vi "Double FFT Mesurament RT.vi"() -> ()   [LabVIEW 2014]
uses:
  <vilib>/Platform/TimedLoop/XDataNode/timing_clust.ctl
  <vilib>/Platform/TimedLoop/XDataNode/nitl_modes.ctl
  <vilib>/Platform/TimedLoop/XDataNode/wakeup.ctl
  <vilib>/FPGAPlugInAG/sbRIO-9636/niLvFpga_Open_sbRIO-9636.vi
  <vilib>/rvi/interface/common/dynamic/niFpgaDynamicAddResources.vi
  <vilib>/Utility/error.llb/Error Cluster From Error Code.vi
  <vilib>/rvi/errors/niLvFpgaAdjustHostInterfaceError.vi
  <vilib>/rvi/interface/common/niFpgaWaitOnOcc.vi
  <vilib>/FPGAPlugInAG/Dynamic/niLvFpga_Run_Dynamic.vi
  <vilib>/FPGAPlugInAG/Dynamic/niLvFpga_Abort_Dynamic.vi
  <vilib>/FPGAPlugInAG/Dynamic/niLvFpga_Reset_Dynamic.vi
  <vilib>/FPGAPlugInAG/Dynamic/niLvFpga_Close_Dynamic.vi
  <vilib>/rvi/interface/nirviOpenFPGA/nirviOpenFPGA.xnode
  FPGA Bitfiles/LaserDistanceSen_FPGATarget_DoubleFFTMesuram_r82pz3ZO4sk.lvbitx
  FPGA Target/Test VIs/Double FFT Mesurament Test.vi
  FPGA Bitfiles/LaserDistanceSen_FPGATarget_DoubleFFTMesuram_atjrRfXVdPQ.lvbitx
  FPGA Target/Test VIs/Double FFT Mesurament Test SLOW.vi
  <vilib>/rvi/interface/nirviReadWriteControl/nirviReadWriteControl.xnode
  <vilib>/rvi/interface/nirviMethod/nirviMethod.xnode
  <vilib>/Platform/TimedLoop/XDataNode/XDataNode.xnode
  <vilib>/rvi/interface/nirviCloseFPGA/nirviCloseFPGA.xnode
  <vilib>/FPGAPlugInAG/Dynamic/niLvFpga_ConfigureFifo_Dynamic.vi
  <vilib>/rvi/errors/niLvFpgaMergeErrorWithErrorCode.vi
  <vilib>/FPGAPlugInAG/Dynamic/niLvFpga_StartFifo_Dynamic.vi
  <vilib>/rvi/interface/Simulation/niFpgaSimulationCallBeginRW.vi
  <vilib>/FPGAPlugInAG/Dynamic/niLvFpga_ReadFifo_Dynamic.vi
  <vilib>/Platform/TimedLoop/XDataNode/XDNodeRunTimeDep.lvlib
  NiFpgaLv.dll
panel:
  in  "Sample /Modulation Frequency":enum32{"40MHz/32KHz", "30MHz/24Khz"}(radio)
  out "Det Freq 1 (3-point) 2":dbl(graph)
  out "Det Freq 1":dbl(graph)
  out "Det Freq 2":T1(graph)
  out "Det Freq 2 (3-point)":dbl(graph)
  out "Detected Frequency (Hz) 1 (3-point)":dbl
  out "Detected Frequency (Hz) 2 (3-point)":dbl
  in  "Scale factor":dbl=1.0 format="%#_13g"
  out "Mean Noise 2":dbl
  out "Mean Noise 1":dbl
  in  "tieni premuto per":i32=1
  out "Mean Frequency":dbl
  out "Velocity (m/s)":dbl
  out "Distance (m)":dbl
  in  "Triangolo dritto?":bool
  out "Detected Frequency (Hz) 2":dbl
  out "Detected Frequency (Hz) 1":dbl
  out "Interpolate Bin 2":dbl
  out "Interpolate Bin 1":dbl
  out "Check Delta Amp Ok? 2":bool
  out "Check Delta Amp Ok? 1":bool
  out "Delta difference % 2":dbl
  out "Delta difference % 1":dbl
  in  "Max Delta Difference bin % 2":dbl=10.0
  in  "Max Delta Difference bin % 1":dbl=10.0
  out "Check Amp 2 Ok?":bool
  out "Check Amp Ok?":bool
  in  "Threshold Amp 2":dbl=5500.0
  in  "Threshold Amp 1":dbl=5500.0
  out "Prev Max Bin 2":i32
  out "Max Bin 2":i32
  out "Succ Max Bin 2":i32
  out "Prev Max Amp 2":dbl
  out "Max Amp 2":dbl
  out "Succ Max Amp 2":dbl
  out "Succ Max Amp":dbl
  out "Max Amp":dbl
  out "Prev Max Amp":dbl
  out "Succ Max Bin":i32
  out "Max Bin":i32
  out "Prev Max Bin":i32
  in  "stop":bool
  in  "Initial Latency points":u32(slide) scale=0.0..1249.0
  out "Second FFT (bin)":dbl[](graph)
  out "Second Signal (points) - Rising Triangular":dbl[](graph)
  out "Elements Remaining FFT":u32
  out "Elements Remaining Signal":u32
  out "First FFT (bin)":dbl[](graph)
  out "First Signal (points) - Falling Triangular":dbl[](graph)
  in  "Snapshot":bool
  in  "Windowing":T2(ring)
  in  "first bin":i32=5
  in  "last bin":i32=255
  in  "lower limit 2":u32(slide)=738 scale=625.0..738.0
  in  "lower limit 1":u32(slide)=113 scale=0.0..113.0
  # "OFFLINE parameters"
  # "WARNING:\nOnce pressed wait untill the end of operation"
  # "Max Detection FFT bin range"
  # "Bin \nDetection"
  # "(2*Max_rumore=2*2700)"
  # "Bin Amplitude\n      CHECK"
  # "(2*Max_rumore=2*2700)"
  # "Bin difference\n     CHECK"
  # "Bin interpolation"
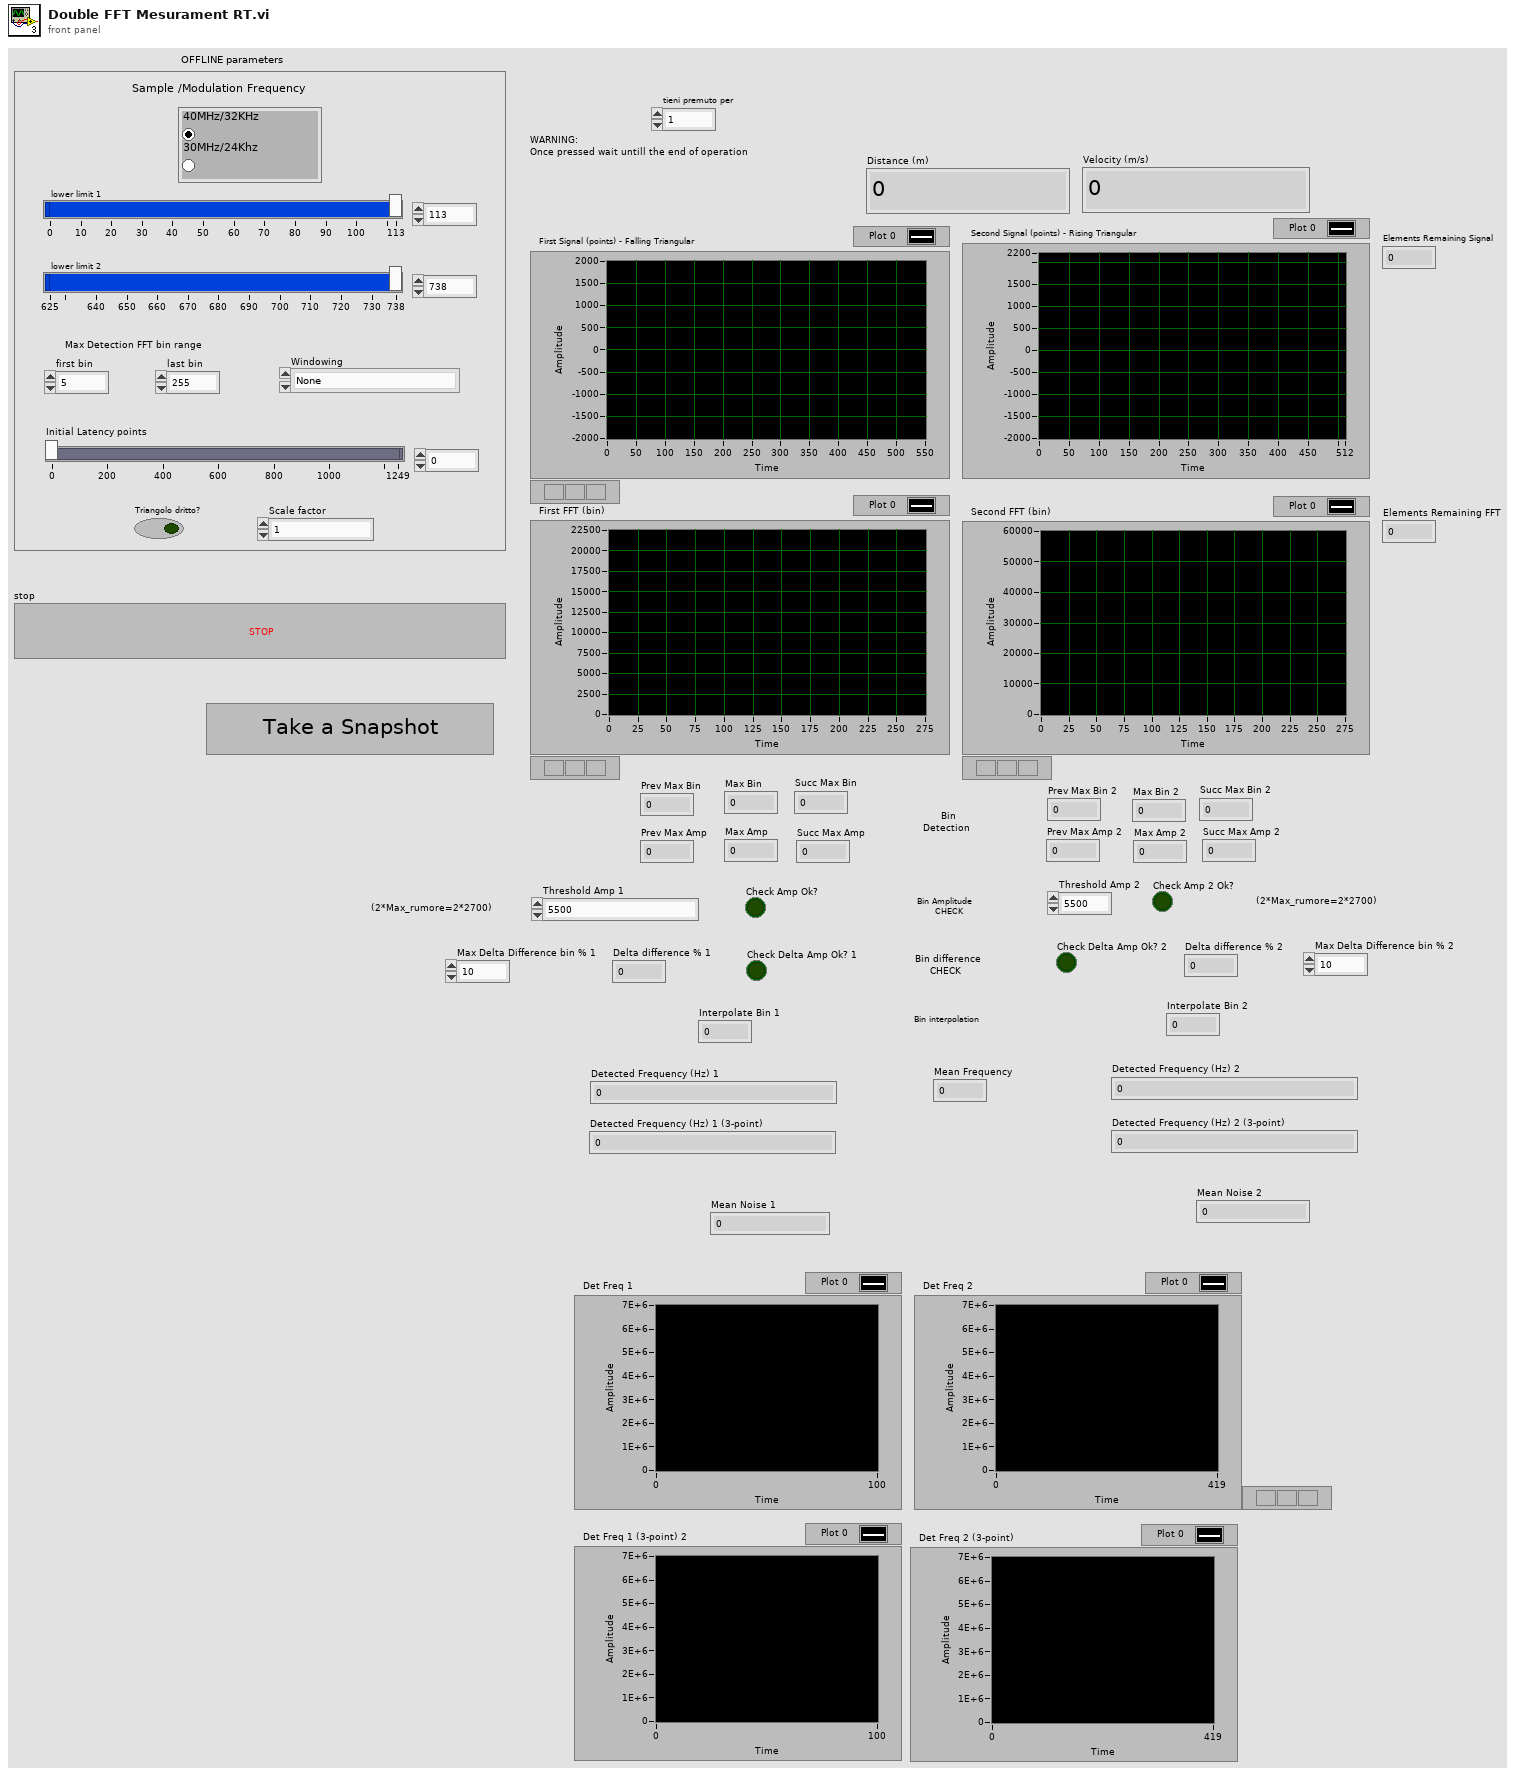
[diagram p1: front panel]
types:
  T1 = cluster{"Delta difference %":dbl, "Detected Frequency (Hz)":dbl}
  T2 = enum16{"None", "Hanning", "Hamming", "Blackman", "Blackman-Harris"}
  T3 = typedef "XDNodeRunTimeDep.lvlib/timing_clust.ctl" = cluster{"Expected End [f-1]":u64, "Actual End [f-1]":u64, "Finished Late? [f-1]":bool, "Expected End [i-1]":u64, "Actual End [i-1]":u64, "Finished Late? [i-1]":bool, "Expected Start [i]":u64, "Actual Start [i]":u64, "Expected Start [f]":u64, "Actual Start [f]":u64, "Source Name":string, "Structure Name":string, "Period":i64, "Deadline":i64, "Offset":i64, "Start":i64, "Priority":i32, "Timeout":i32, "Mode":T4, "Wakeup Reason":T5, "Error":errorcluster, "Source Type":string, "Secondary Source Type":string, "Global End Time":u64, "Global Start Time":u64, "Frame Duration":u64, "Iteration Duration":u64, "Assigned CPU":i32, "I/O Scan Engine Mode":u32}
  T4 = typedef "XDNodeRunTimeDep.lvlib/nitl_modes.ctl" = enum32{"No Change", "Process missed periods, maintain original phase", "Discard missed periods, maintain original phase", "Process missed periods, ignore original phase", "Discard missed periods, ignore original phase"}
  T5 = typedef "XDNodeRunTimeDep.lvlib/wakeup.ctl" = enum32{"Normal", "Aborted", "Asynchronous wakeup", "Timing source error", "Timed loop error", "Timeout"}
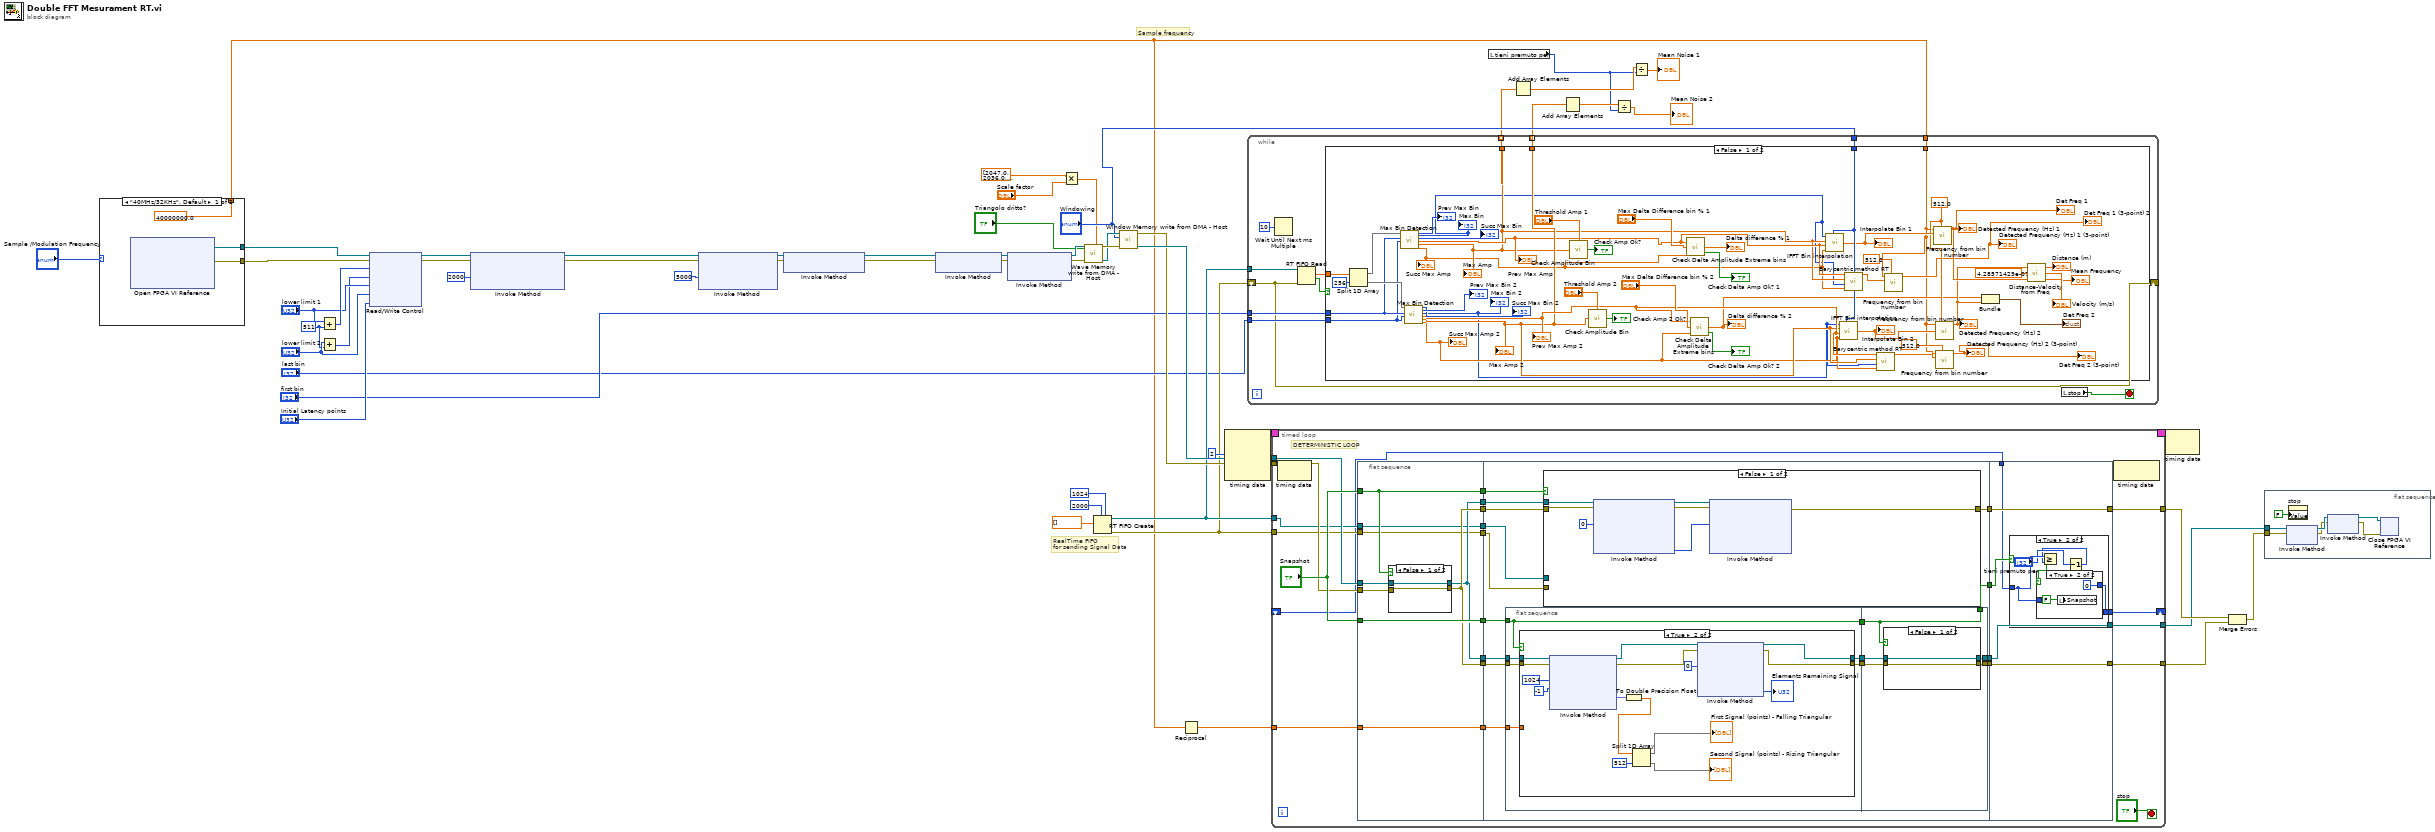
[diagram p0: block diagram]
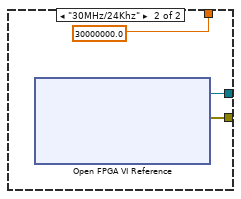
[diagram p2: hidden frame]
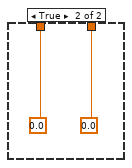
[diagram p3: hidden frame]
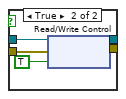
[diagram p4: hidden frame]
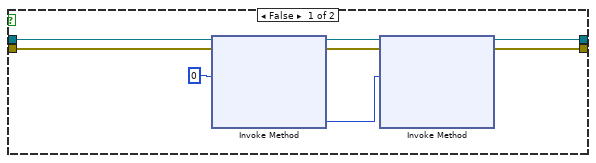
[diagram p5: hidden frame]
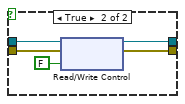
[diagram p6: hidden frame]
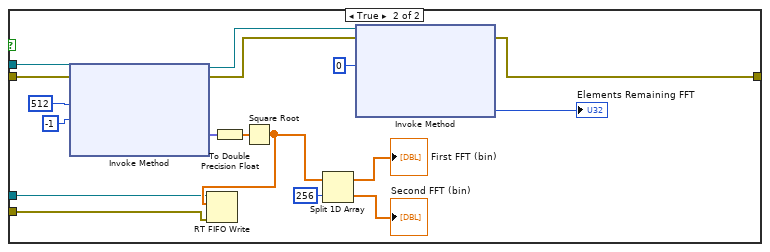
[diagram p7: hidden frame]
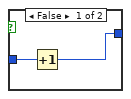
[diagram p9: hidden frame]
diagram:
  w51 = u32 511 ("y")
  # "Sample frequency"
  # "RealTime FIFO \nfor sending Signal Data"
  n1 = case shown="\"40MHz/32KHz\", Default" "Sample /Modulation Frequency" {
    tunnel: [w58 w61] -> w50
    tunnel: [w57 w60] -> w49
    tunnel: [40000000.0 30000000.0] -> w1
    frame "40MHz/32KHz", Default {
      n2 = xnode "Open FPGA VI Reference"() -> ("FPGA VI Reference Out"=w58:refnum<k20>, "error out"=w57:errorcluster)  [unwired: 2 in]
    }
    frame "30MHz/24Khz" {
      n3 = xnode "Open FPGA VI Reference"() -> ("FPGA VI Reference Out"=w61:refnum<k20>, "error out"=w60:errorcluster)  [unwired: 2 in]
    }
  }
  n4 = Add(x="lower limit 1", y=w51) -> (x+y=w55:u32)
  n5 = Add(x="lower limit 2", y=w51) -> (x+y=w53:u32)
  n6 = xnode "Read/Write Control"("FPGA VI Reference In"=w50, "error in"=w49, "upper limit 1"=w55, "upper limit 2"=w53, "lower limit 1"="lower limit 1", "lower limit 2"="lower limit 2", "Latency points"="Initial Latency points") -> ("FPGA VI Reference Out"=w46:refnum<k20>, "error out"=w45:errorcluster)
  n7 = xnode "Invoke Method"("FPGA VI Reference In"=w46, "error in"=w45, "Requested Depth"=u32 2000) -> ("FPGA VI Reference Out"=w24:refnum<k20>, "error out"=w25:errorcluster)  [unwired: 1 out]
  n8 = xnode "Invoke Method"("FPGA VI Reference In"=w24, "error in"=w25, "Requested Depth"=u32 5000) -> ("FPGA VI Reference Out"=w36:refnum<k20>, "error out"=w37:errorcluster)  [unwired: 1 out]
  n9 = xnode "Invoke Method"("FPGA VI Reference In"=w36, "error in"=w37) -> ("FPGA VI Reference Out"=w22:refnum<k20>, "error out"=w23:errorcluster)
  n10 = xnode "Invoke Method"("FPGA VI Reference In"=w22, "error in"=w23) -> ("FPGA VI Reference Out"=w34:refnum<k20>, "error out"=w35:errorcluster)
  n11 = xnode "Invoke Method"("FPGA VI Reference In"=w34, "error in"=w35) -> ("FPGA VI Reference Out"=w40:refnum<k20>, "error out"=w39:errorcluster)  [unwired: 1 in]
  n12 = Multiply(x=dbl[] [2047.0, 2036.0, 2024.0, 2013.0, 2002.0, 1990.0, 1979.0, 1968.0, 1956.0, 1945.0, 1934.0, 1923.0, 1912.0, 1900.0, 1889.0, 1878.0, 1867.0, 1856.0, 1845.0, 1833.0, 1822.0, 1811.0, 1800.0, 1789.0, 1778.0, 1767.0, 1756.0, 1745.0, 1734.0, 1723.0, 1712.0, 1702.0, 1691.0, 1680.0, 1669.0, 1658.0, 1647.0, 1636.0, 1626.0, 1615.0, 1604.0, 1593.0, 1583.0, 1572.0, 1561.0, 1550.0, 1540.0, 1529.0, 1518.0, 1508.0, 1497.0, 1487.0, 1476.0, 1465.0, 1455.0, 1444.0, 1434.0, 1423.0, 1413.0, 1402.0, 1392.0, 1381.0, 1371.0, 1360.0, 1350.0, 1340.0, 1329.0, 1319.0, 1309.0, 1298.0, 1288.0, 1278.0, 1267.0, 1257.0, 1247.0, 1237.0, 1226.0, 1216.0, 1206.0, 1196.0, 1186.0, 1176.0, 1165.0, 1155.0, 1145.0, 1135.0, 1125.0, 1115.0, 1105.0, 1095.0, 1085.0, 1075.0, 1065.0, 1055.0, 1045.0, 1035.0, 1025.0, 1015.0, 1006.0, 996.0, 986.0, 976.0, 966.0, 956.0, 947.0, 937.0, 927.0, 917.0, 908.0, 898.0, 888.0, 879.0, 869.0, 859.0, 850.0, 837.0, 826.0, 816.0, 804.0, 796.0, 788.0, 778.0, 769.0, 758.0, 750.0, 743.0, 733.0, 724.0, 717.0, 709.0, 701.0, 693.0, 686.0, 677.0, 669.0, 661.0, 653.0, 645.0, 638.0, 630.0, 622.0, 615.0, 607.0, 599.0, 592.0, 583.0, 576.0, 569.0, 561.0, 554.0, 547.0, 539.0, 532.0, 525.0, 518.0, 509.0, 501.0, 492.0, 486.0, 478.0, 471.0, 463.0, 456.0, 450.0, 442.0, 435.0, 429.0, 421.0, 415.0, 408.0, 401.0, 394.0, 388.0, 381.0, 375.0, 368.0, 361.0, 355.0, 349.0, 342.0, 336.0, 330.0, 323.0, 317.0, 311.0, 304.0, 298.0, 292.0, 286.0, 279.0, 273.0, 267.0, 261.0, 255.0, 249.0, 242.0, 236.0, 230.0, 224.0, 218.0, 212.0, 206.0, 200.0, 194.0, 187.0, 181.0, 175.0, 169.0, 163.0, 157.0, 150.0, 144.0, 138.0, 132.0, 125.0, 119.0, 113.0, 107.0, 101.0, 95.0, 88.0, 82.0, 77.0, 71.0, 65.0, 59.0, 53.0, 47.0, 41.0, 35.0, 29.0, 23.0, 18.0, 11.0, 6.0, 0.0, -6.0, -12.0, -18.0, -23.0, -29.0, -35.0, -41.0, -47.0, -52.0, -58.0, -64.0, -69.0, -75.0, -81.0, -87.0, -92.0, -98.0, -104.0, -109.0, -115.0, -121.0, -126.0, -132.0, -138.0, -144.0, -149.0, -155.0, -161.0, -166.0, -172.0, -177.0, -183.0, -189.0, -194.0, -200.0, -205.0, -211.0, -216.0, -222.0, -227.0, -233.0, -238.0, -244.0, -249.0, -255.0, -260.0, -266.0, -271.0, -277.0, -283.0, -288.0, -294.0, -299.0, -304.0, -310.0, -315.0, -321.0, -326.0, -331.0, -337.0, -342.0, -348.0, -353.0, -358.0, -364.0, -369.0, -375.0, -380.0, -385.0, -391.0, -396.0, -402.0, -407.0, -413.0, -418.0, -423.0, -429.0, -434.0, -439.0, -445.0, -450.0, -456.0, -461.0, -466.0, -472.0, -477.0, -483.0, -488.0, -493.0, -499.0, -504.0, -510.0, -515.0, -520.0, -526.0, -531.0, -537.0, -542.0, -548.0, -553.0, -558.0, -564.0, -569.0, -574.0, -580.0, -585.0, -590.0, -596.0, -601.0, -606.0, -612.0, -617.0, -622.0, -628.0, -633.0, -638.0, -644.0, -649.0, -654.0, -660.0, -665.0, -670.0, -676.0, -681.0, -686.0, -692.0, -697.0, -702.0, -708.0, -713.0, -718.0, -723.0, -729.0, -734.0, -739.0, -744.0, -750.0, -755.0, -760.0, -765.0, -771.0, -776.0, -781.0, -786.0, -792.0, -797.0, -802.0, -807.0, -812.0, -818.0, -823.0, -828.0, -833.0, -839.0, -844.0, -849.0, -854.0, -859.0, -865.0, -870.0, -875.0, -880.0, -885.0, -891.0, -896.0, -901.0, -906.0, -911.0, -916.0, -922.0, -927.0, -932.0, -937.0, -943.0, -948.0, -953.0, -958.0, -963.0, -969.0, -974.0, -979.0, -984.0, -989.0, -995.0, -1000.0, -1005.0, -1010.0, -1015.0, -1021.0, -1026.0, -1031.0, -1036.0, -1041.0, -1047.0, -1052.0, -1057.0, -1062.0, -1067.0, -1073.0, -1078.0, -1083.0, -1088.0, -1093.0, -1099.0, -1104.0, -1109.0, -1114.0, -1119.0, -1124.0, -1130.0, -1135.0, -1140.0, -1145.0, -1150.0, -1156.0, -1161.0, -1166.0, -1171.0, -1176.0, -1182.0, -1187.0, -1192.0, -1197.0, -1202.0, -1207.0, -1213.0, -1218.0, -1223.0, -1228.0, -1233.0, -1238.0, -1244.0, -1249.0, -1254.0, -1259.0, -1264.0, -1269.0, -1275.0, -1280.0, -1285.0, -1290.0, -1295.0, -1300.0, -1305.0, -1311.0, -1316.0, -1321.0, -1326.0, -1331.0, -1336.0, -1342.0, -1347.0, -1352.0, -1357.0, -1362.0, -1367.0, -1372.0, -1378.0, -1383.0, -1388.0, -1393.0, -1398.0, -1403.0, -1408.0, -1414.0, -1419.0, -1424.0, -1429.0, -1434.0, -1439.0, -1444.0, -1450.0, -1455.0, -1460.0, -1465.0, -1470.0, -1475.0, -1480.0, -1486.0, -1491.0, -1496.0, -1501.0, -1506.0, -1511.0, -1516.0, -1522.0, -1527.0, -1532.0, -1537.0, -1542.0, -1547.0, -1552.0, -1558.0, -1563.0, -1568.0, -1573.0, -1578.0, -1583.0, -1588.0, -1593.0, -1599.0, -1604.0, -1609.0, -1614.0, -1619.0, -1624.0, -1629.0, -1634.0, -1640.0, -1645.0, -1650.0, -1655.0, -1660.0, -1665.0, -1670.0, -1675.0, -1681.0, -1686.0, -1691.0, -1696.0, -1701.0, -1706.0, -1711.0, -1716.0, -1722.0, -1727.0, -1732.0, -1737.0, -1742.0, -1747.0, -1752.0, -1757.0, -1762.0, -1768.0, -1773.0, -1778.0, -1783.0, -1788.0, -1793.0, -1798.0, -1803.0, -1808.0, -1814.0, -1819.0, -1824.0, -1829.0, -1834.0, -1839.0, -1844.0, -1849.0, -1854.0, -1859.0, -1865.0, -1870.0, -1875.0, -1880.0, -1885.0, -1890.0, -1895.0, -1900.0, -1905.0, -1911.0, -1916.0, -1921.0, -1926.0, -1931.0, -1936.0, -1941.0, -1946.0, -1951.0, -1956.0, -1961.0, -1967.0, -1972.0, -1977.0, -1982.0, -1987.0, -1992.0, -1997.0, -2002.0, -2007.0, -2012.0, -2017.0, -2023.0, -2028.0, -2033.0, -2038.0, -2043.0, -2048.0, -2047.0, -2034.0, -2021.0, -2009.0, -1996.0, -1983.0, -1970.0, -1957.0, -1945.0, -1932.0, -1919.0, -1907.0, -1894.0, -1881.0, -1869.0, -1856.0, -1844.0, -1831.0, -1819.0, -1806.0, -1794.0, -1781.0, -1769.0, -1757.0, -1744.0, -1732.0, -1719.0, -1707.0, -1695.0, -1682.0, -1670.0, -1658.0, -1646.0, -1634.0, -1621.0, -1609.0, -1597.0, -1585.0, -1573.0, -1561.0, -1549.0, -1537.0, -1525.0, -1513.0, -1501.0, -1489.0, -1477.0, -1465.0, -1453.0, -1441.0, -1429.0, -1417.0, -1405.0, -1394.0, -1382.0, -1370.0, -1358.0, -1347.0, -1335.0, -1323.0, -1312.0, -1300.0, -1288.0, -1277.0, -1265.0, -1254.0, -1242.0, -1231.0, -1219.0, -1208.0, -1196.0, -1185.0, -1173.0, -1162.0, -1150.0, -1139.0, -1128.0, -1116.0, -1105.0, -1094.0, -1083.0, -1071.0, -1060.0, -1049.0, -1038.0, -1027.0, -1015.0, -1004.0, -993.0, -982.0, -971.0, -960.0, -949.0, -938.0, -927.0, -916.0, -905.0, -894.0, -883.0, -873.0, -862.0, -851.0, -840.0, -829.0, -819.0, -808.0, -797.0, -786.0, -776.0, -765.0, -754.0, -744.0, -733.0, -722.0, -712.0, -697.0, -685.0, -674.0, -661.0, -652.0, -643.0, -632.0, -622.0, -610.0, -602.0, -594.0, -583.0, -574.0, -566.0, -558.0, -550.0, -542.0, -534.0, -525.0, -516.0, -507.0, -499.0, -491.0, -483.0, -475.0, -467.0, -459.0, -451.0, -443.0, -435.0, -426.0, -419.0, -411.0, -404.0, -396.0, -388.0, -381.0, -373.0, -366.0, -359.0, -349.0, -341.0, -331.0, -325.0, -317.0, -309.0, -301.0, -295.0, -288.0, -280.0, -273.0, -266.0, -259.0, -252.0, -246.0, -239.0, -231.0, -225.0, -219.0, -212.0, -205.0, -199.0, -192.0, -186.0, -180.0, -173.0, -167.0, -161.0, -155.0, -148.0, -142.0, -136.0, -130.0, -124.0, -118.0, -112.0, -106.0, -100.0, -94.0, -88.0, -82.0, -76.0, -70.0, -64.0, -58.0, -52.0, -46.0, -40.0, -34.0, -28.0, -21.0, -15.0, -9.0, -3.0, 2.0, 9.0, 15.0, 21.0, 27.0, 33.0, 39.0, 45.0, 51.0, 57.0, 63.0, 69.0, 75.0, 81.0, 86.0, 92.0, 98.0, 103.0, 110.0, 116.0, 121.0, 127.0, 133.0, 138.0, 144.0, 149.0, 155.0, 161.0, 166.0, 172.0, 177.0, 183.0, 189.0, 194.0, 200.0, 205.0, 211.0, 216.0, 221.0, 227.0, 232.0, 238.0, 243.0, 249.0, 254.0, 259.0, 265.0, 270.0, 276.0, 281.0, 286.0, 292.0, 297.0, 303.0, 308.0, 314.0, 319.0, 324.0, 329.0, 335.0, 340.0, 345.0, 351.0, 356.0, 361.0, 366.0, 371.0, 377.0, 382.0, 387.0, 392.0, 397.0, 403.0, 408.0, 413.0, 418.0, 423.0, 429.0, 434.0, 439.0, 444.0, 449.0, 454.0, 459.0, 464.0, 469.0, 474.0, 479.0, 484.0, 489.0, 494.0, 499.0, 504.0, 509.0, 514.0, 520.0, 525.0, 530.0, 535.0, 540.0, 545.0, 550.0, 555.0, 560.0, 565.0, 570.0, 575.0, 580.0, 585.0, 590.0, 595.0, 600.0, 605.0, 610.0, 615.0, 620.0, 625.0, 630.0, 636.0, 641.0, 646.0, 651.0, 656.0, 661.0, 666.0, 671.0, 676.0, 681.0, 686.0, 691.0, 696.0, 701.0, 706.0, 711.0, 716.0, 721.0, 726.0, 731.0, 736.0, 741.0, 746.0, 751.0, 756.0, 761.0, 765.0, 770.0, 775.0, 780.0, 785.0, 790.0, 795.0, 800.0, 805.0, 810.0, 815.0, 820.0, 825.0, 829.0, 834.0, 839.0, 844.0, 849.0, 854.0, 859.0, 864.0, 868.0, 873.0, 878.0, 883.0, 888.0, 893.0, 897.0, 902.0, 907.0, 912.0, 917.0, 921.0, 926.0, 931.0, 936.0, 941.0, 945.0, 950.0, 955.0, 960.0, 965.0, 969.0, 974.0, 979.0, 984.0, 988.0, 993.0, 998.0, 1003.0, 1007.0, 1012.0, 1017.0, 1022.0, 1027.0, 1031.0, 1036.0, 1041.0, 1046.0, 1051.0, 1055.0, 1060.0, 1065.0, 1070.0, 1075.0, 1079.0, 1084.0, 1089.0, 1094.0, 1098.0, 1103.0, 1108.0, 1113.0, 1118.0, 1122.0, 1127.0, 1132.0, 1137.0, 1141.0, 1146.0, 1151.0, 1156.0, 1161.0, 1165.0, 1170.0, 1175.0, 1180.0, 1184.0, 1189.0, 1194.0, 1199.0, 1204.0, 1208.0, 1213.0, 1218.0, 1223.0, 1227.0, 1232.0, 1237.0, 1242.0, 1246.0, 1251.0, 1256.0, 1261.0, 1265.0, 1270.0, 1275.0, 1280.0, 1284.0, 1289.0, 1294.0, 1299.0, 1303.0, 1308.0, 1313.0, 1318.0, 1322.0, 1327.0, 1332.0, 1336.0, 1341.0, 1346.0, 1351.0, 1355.0, 1360.0, 1365.0, 1370.0, 1374.0, 1379.0, 1384.0, 1388.0, 1393.0, 1398.0, 1403.0, 1407.0, 1412.0, 1417.0, 1421.0, 1426.0, 1431.0, 1436.0, 1440.0, 1445.0, 1450.0, 1454.0, 1459.0, 1464.0, 1469.0, 1473.0, 1478.0, 1483.0, 1487.0, 1492.0, 1497.0, 1502.0, 1506.0, 1511.0, 1516.0, 1520.0, 1525.0, 1530.0, 1535.0, 1539.0, 1544.0, 1549.0, 1553.0, 1558.0, 1563.0, 1567.0, 1572.0, 1577.0, 1582.0, 1586.0, 1591.0, 1596.0, 1600.0, 1605.0, 1610.0, 1614.0, 1619.0, 1624.0, 1628.0, 1633.0, 1638.0, 1643.0, 1647.0, 1652.0, 1657.0, 1661.0, 1666.0, 1671.0, 1675.0, 1680.0, 1685.0, 1689.0, 1694.0, 1699.0, 1703.0, 1708.0, 1713.0, 1717.0, 1722.0, 1727.0, 1731.0, 1736.0, 1741.0, 1746.0, 1750.0, 1755.0, 1760.0, 1764.0, 1769.0, 1774.0, 1778.0, 1783.0, 1788.0, 1792.0, 1797.0, 1802.0, 1806.0, 1811.0, 1816.0, 1820.0, 1825.0, 1830.0, 1834.0, 1839.0, 1844.0, 1848.0, 1853.0, 1858.0, 1862.0, 1867.0, 1871.0, 1876.0, 1881.0, 1885.0, 1890.0, 1895.0, 1899.0, 1904.0, 1909.0, 1913.0, 1918.0, 1923.0, 1927.0, 1932.0, 1937.0, 1941.0, 1946.0, 1951.0, 1955.0, 1960.0, 1965.0, 1969.0, 1974.0, 1978.0, 1983.0, 1988.0, 1992.0, 1997.0, 2002.0, 2006.0, 2011.0, 2016.0, 2020.0, 2025.0, 2029.0, 2034.0, 2039.0, 2043.0, 2048.0] ("Complete SkewTri"), y="Scale factor") -> (x*y=w4:dbl[])
  n13 = call "Wave Memory write from DMA - Host.vi"("Custom Triangular Signal (fal-ris)"=w4, "Triangolo dritto?"="Triangolo dritto?", "error in"=w39, "FPGA VI Reference In"=w40) -> ("FPGA VI Reference Out"=w27:refnum<k20>, "error out"=w38:errorcluster)  [unwired: 5 in, 1 out]
  n14 = RT FIFO Create(1:dbl[] [] ("double precision float"), 4:u32 2000 ("size (10)"), 6:u32 1024 ("elements in array (1)")) -> (8:w18:refnum<k33>, 11:w17:errorcluster)  [unwired: 5 in, 1 out]
  n15 = call "Window Memory write from DMA - Host.vi"("error in"=w38, "Enum"="Windowing", "FPGA VI Reference In"=w27) -> ("FPGA VI Reference Out"=w48:refnum<k20>, "error out"=w47:errorcluster)  [unwired: 5 in, 2 out]
  n16 = Reciprocal(x=w1) -> (1/x=w41:dbl)
  n17 = node-c288(i64 2 ("Period")) -> (w33:T3)  [unwired: 3 in]
  n18 = while {
    tunnel: w18 -> [w72]
    shift-right: [w65] -> _
    shift-left: w17 -> [w65]
    tunnel: "first bin" -> [w70]
    tunnel: "last bin" -> [w69]
    tunnel: "Windowing" -> [w66]
    tunnel: [w64] -> w12 mode=indexing
    tunnel: [w63] -> w11 mode=indexing
    tunnel: w1 -> [w62]
    stop <- w73 stop-if-true
    n19 = Wait Until Next ms Multiple(millisecond multiple=u32 10) -> ()  [unwired: 1 out]
    n20 = RT FIFO Read(0:w72, 3:w65) -> (9:w71:dbl[], 10:w67:bool)  [unwired: 2 in, 3 out]
    n21 = case shown="False" w67 {
      tunnel: w71 -> [w118 _]
      tunnel: w70 -> [w115 _]
      tunnel: w69 -> [w114 _]
      tunnel: w66 -> [w100 _]
      tunnel: [w87 0.0 ("Max Amp")] -> w64
      tunnel: [w91 0.0 ("Prev Max Amp")] -> w63
      tunnel: w62 -> [w74 _]
      frame False {
        w97 = 512.0 ("FFT size")
        n22 = Split 1D Array(array=w118, index=256) -> (first subarray=w117:dbl[], second subarray=w116:dbl[])
        n23 = call "Max Bin Detection.vi"("FFT Array"=w117, "Init Discard Bins"=w115, "Last Discard Bins"=w114) -> ("Prev Max Bin"=→"Prev Max Bin":i32, "Max Bin"=w85:i32, "Succ Max Bin"=→"Succ Max Bin":i32, "Prev Max Amp"=w88:dbl, "Max Amp"=w87:dbl, "Succ Max Amp"=w86:dbl)  [unwired: 11 in]
        "Max Bin" <- w85
        "Prev Max Amp" <- w88
        "Max Amp" <- w87
        "Succ Max Amp" <- w86
        n24 = call "Max Bin Detection.vi"("FFT Array"=w116, "Init Discard Bins"=w115, "Last Discard Bins"=w114) -> ("Prev Max Bin"=→"Prev Max Bin 2":i32, "Max Bin"=w89:i32, "Succ Max Bin"=→"Succ Max Bin 2":i32, "Prev Max Amp"=w92:dbl, "Max Amp"=w91:dbl, "Succ Max Amp"=w90:dbl)  [unwired: 11 in]
        "Max Bin 2" <- w89
        "Prev Max Amp 2" <- w92
        "Max Amp 2" <- w91
        "Succ Max Amp 2" <- w90
        n25 = call "Check Amplitude Bin.vi"("Threshold Amp"="Threshold Amp 1", "Max Amp"=w87) -> ("Check Amp Ok?"=→"Check Amp Ok?":bool)  [unwired: 2 in]
        n26 = call "Check Amplitude Bin.vi"("Threshold Amp"="Threshold Amp 2", "Max Amp"=w91) -> ("Check Amp Ok?"=→"Check Amp 2 Ok?":bool)  [unwired: 2 in]
        n27 = call "Check Delta Amplitude Extreme bins.vi"("Succ Max Amp"=w86, "Max Difference %"="Max Delta Difference bin % 1", "Prev Max Amp"=w88) -> ("Check Delta Amp Ok?"=→"Check Delta Amp Ok? 1":bool, "Delta difference %"=→"Delta difference % 1":dbl)  [unwired: 1 in]
        n28 = call "Check Delta Amplitude Extreme bins.vi"("Succ Max Amp"=w90, "Max Difference %"="Max Delta Difference bin % 2", "Prev Max Amp"=w92) -> ("Check Delta Amp Ok?"=→"Check Delta Amp Ok? 2":bool, "Delta difference %"=w75:dbl)  [unwired: 1 in]
        "Delta difference % 2" <- w75
        n29 = call "IFFT Bin interpolation.vi"("Max Bin"=w85, "Max Amp"=w87, "Prev Max Amp"=w88, "Succ Max Amp"=w86, "Windowing"=w100) -> ("Interpolate Bin"=w98:dbl)
        "Interpolate Bin 1" <- w98
        n30 = call "IFFT Bin interpolation.vi"("Max Bin"=w89, "Max Amp"=w91, "Prev Max Amp"=w92, "Succ Max Amp"=w90, "Windowing"=w100) -> ("Interpolate Bin"=w99:dbl)
        "Interpolate Bin 2" <- w99
        n31 = call "Barycentric method RT.vi"("Next Amp"=w86, "Max Bin"=w85, "Max Amp"=w87, "Prev Amp"=w88) -> ("Bin"=w82:dbl)  [unwired: 7 in]
        n32 = call "Barycentric method RT.vi"("Next Amp"=w90, "Max Bin"=w89, "Max Amp"=w91, "Prev Amp"=w92) -> ("Bin"=w84:dbl)  [unwired: 7 in]
        n33 = call "Frequency from bin number.vi"("FFT size"=512.0, "Bin number"=w82, "Sample Rate (S/s)"=w74) -> ("Detected Frequency (Hz)"=→"Detected Frequency (Hz) 1 (3-point)" →"Det Freq 1 (3-point) 2":dbl)  [unwired: 8 in]
        n34 = call "Frequency from bin number.vi"("FFT size"=w97, "Bin number"=w98, "Sample Rate (S/s)"=w74) -> ("Detected Frequency (Hz)"=w79:dbl)  [unwired: 8 in]
        "Detected Frequency (Hz) 1" <- w79
        "Det Freq 1" <- w79
        n35 = call "Frequency from bin number.vi"("FFT size"=w97, "Bin number"=w99, "Sample Rate (S/s)"=w74) -> ("Detected Frequency (Hz)"=w76:dbl)  [unwired: 8 in]
        "Detected Frequency (Hz) 2" <- w76
        n36 = call "Frequency from bin number.vi"("FFT size"=512.0, "Bin number"=w84, "Sample Rate (S/s)"=w74) -> ("Detected Frequency (Hz)"=→"Detected Frequency (Hz) 2 (3-point)" →"Det Freq 2 (3-point)":dbl)  [unwired: 8 in]
        n37 = Bundle("Delta difference %"=w75, "Detected Frequency (Hz)"=w76) -> (→"Det Freq 2":T1)  [unwired: 1 in]
        n38 = call "Distance-Velocity from Freq.vi"("freq_rising"=w76, "Empirical Distance Costant"=4.28571429e-07, "freq_falling"=w79) -> ("Distance (m)"=→"Distance (m)":dbl, "Mean Frequency"=→"Mean Frequency":dbl, "Velocity (m/s)"=→"Velocity (m/s)":dbl)  [unwired: 2 in]
      }
      frame True {
      }
    }
    n39 = local read "stop"() -> (w73:bool)
  }
  n40 = timed-loop {
    tunnel: w48 -> [w141]
    tunnel: w47 -> [w142]
    tunnel: [w144] -> w30
    tunnel: w41 -> [w146]
    tunnel: [w145] -> w29
    timing: w33 -> [_]
    timing-out: [_] -> w32
    tunnel: [w129] -> w26
    tunnel: w18 -> [w127]
    tunnel: w17 -> [w124]
    shift-right: [w123] -> _
    shift-left: _ -> [w122]
    stop <- "stop" stop-if-true
    # "DETERMINISTIC LOOP"
    n41 = node-c288() -> ()  [unwired: 1 in, 1 out]
    n42 = flat-sequence {
      tunnel: w141 -> [w153]
      tunnel: w142 -> [w154]
      tunnel: "Snapshot" -> [w151]
      tunnel: "Snapshot" -> [w156]
      tunnel: w146 -> [w157]
      tunnel: [w155] -> w140
      tunnel: [w157] -> w139
      tunnel: [w156] -> w138
      tunnel: [w151] -> w137
      tunnel: [w155] -> w136
      tunnel: [w152] -> w135
      tunnel: [w152] -> w134
      tunnel: w127 -> [w150]
      tunnel: [w150] -> w126
      tunnel: [w149] -> w125
      tunnel: w124 -> [w149]
      tunnel: w140 -> [w176]
      tunnel: w139 -> [w175]
      tunnel: w138 -> [w169]
      tunnel: w137 -> [w172]
      tunnel: w136 -> [w171]
      tunnel: w135 -> [w170]
      tunnel: w134 -> [w177]
      tunnel: [w174] -> w133
      tunnel: [w173] -> w132
      tunnel: [w168] -> w131
      tunnel: [w167] -> w128
      tunnel: w126 -> [w166]
      tunnel: w125 -> [w165]
      tunnel: [w250] -> w144
      tunnel: [w251] -> w145
      tunnel: w133 -> [w251]
      tunnel: w132 -> [w250]
      tunnel: w131 -> [w248]
      tunnel: [w249] -> w129
      tunnel: w128 -> [w249]
      tunnel: [w247] -> w123
      tunnel: w122 -> [w246]
      frame #0 {
        n43 = case shown="False" w151 {
          tunnel: [w158 w163] -> w155
          tunnel: w154 -> [w158 w162]
          tunnel: w153 -> [w159 w161]
          tunnel: [w159 w160] -> w152
          frame False {
          }
          frame True {
            n44 = xnode "Read/Write Control"("FPGA VI Reference In"=w161, "error in"=w162, "snapshot"=TRUE) -> ("FPGA VI Reference Out"=w160:refnum<k20>, "error out"=w163:errorcluster)
          }
        }
      }
      frame #1 {
        n45 = flat-sequence {
          tunnel: w177 -> [w186]
          tunnel: w176 -> [w185]
          tunnel: w175 -> [w184]
          tunnel: w169 -> [w181]
          tunnel: [w183] -> w180
          tunnel: [w182] -> w179
          tunnel: [w181] -> w178
          tunnel: [w212] -> w173
          tunnel: w180 -> [w214]
          tunnel: w179 -> [w213]
          tunnel: w178 -> [w211]
          tunnel: [w211] -> w168
          tunnel: [w210] -> w167
          frame #0 {
            n46 = case shown="True" w181 {
              tunnel: w186 -> [w193 w209]
              tunnel: w185 -> [w191 w208]
              tunnel: [w190 w201] -> w182
              tunnel: w184 -> [_ _]
              tunnel: [w187 w200] -> w183
              frame False {
                n47 = xnode "Invoke Method"("FPGA VI Reference In"=w193, "error in"=w191, "Number of Elements"=u32 0) -> ("FPGA VI Reference Out"=w189:refnum<k20>, "error out"=w188:errorcluster, "Elements Remaining"=w192:u32)  [unwired: 1 in, 1 out]
                n48 = xnode "Invoke Method"("FPGA VI Reference In"=w189, "error in"=w188, "Number of Elements"=w192) -> ("FPGA VI Reference Out"=w187:refnum<k20>, "error out"=w190:errorcluster)  [unwired: 1 in, 2 out]
              }
              frame True {
                n49 = xnode "Invoke Method"("FPGA VI Reference In"=w209, "error in"=w208, "Number of Elements"=u32 1024, "Timeout (ms)"=-1) -> ("FPGA VI Reference Out"=w203:refnum<k20>, "error out"=w202:errorcluster, "Data"=w205:fxp<+/-,12,12>[])  [unwired: 1 out]
                n50 = To Double Precision Float(number=w205) -> (double precision float=w198:dbl[])
                n51 = Split 1D Array(array=w198, index=512) -> (first subarray=→"First Signal (points) - Falling Triangular":dbl[], second subarray=→"Second Signal (points) - Rising Triangular":dbl[])
                n52 = xnode "Invoke Method"("FPGA VI Reference In"=w203, "error in"=w202, "Number of Elements"=u32 0) -> ("FPGA VI Reference Out"=w200:refnum<k20>, "error out"=w201:errorcluster, "Elements Remaining"=→"Elements Remaining Signal":u32)  [unwired: 1 in, 1 out]
              }
            }
          }
          frame #1 {
            n53 = case shown="False" w211 {
              tunnel: [w216 w219] -> w212
              tunnel: w214 -> [w215 w220]
              tunnel: w213 -> [w216 w218]
              tunnel: [w215 w217] -> w210
              frame False {
              }
              frame True {
                n54 = xnode "Read/Write Control"("FPGA VI Reference In"=w220, "error in"=w218, "snapshot"=FALSE) -> ("FPGA VI Reference Out"=w217:refnum<k20>, "error out"=w219:errorcluster)
              }
            }
          }
        }
        n55 = case shown="False" w172 {
          tunnel: w170 -> [w227 w240]
          tunnel: w171 -> [w224 w241]
          tunnel: [w223 w239] -> w174
          tunnel: w166 -> [_ w230]
          tunnel: w165 -> [_ w229]
          frame False {
            n56 = xnode "Invoke Method"("FPGA VI Reference In"=w227, "error in"=w224, "Number of Elements"=u32 0) -> ("FPGA VI Reference Out"=w225:refnum<k20>, "error out"=w222:errorcluster, "Elements Remaining"=w226:u32)  [unwired: 1 in, 1 out]
            n57 = xnode "Invoke Method"("FPGA VI Reference In"=w225, "error in"=w222, "Number of Elements"=w226) -> ("error out"=w223:errorcluster)  [unwired: 1 in, 3 out]
          }
          frame True {
            n58 = xnode "Invoke Method"("FPGA VI Reference In"=w240, "error in"=w241, "Number of Elements"=u32 512, "Timeout (ms)"=-1) -> ("FPGA VI Reference Out"=w237:refnum<k20>, "error out"=w238:errorcluster, "Data"=w243:fxp<+,44,44>[])  [unwired: 1 out]
            n59 = To Double Precision Float(number=w243) -> (double precision float=w242:dbl[])
            n60 = Square Root(x=w242) -> (sqrt(x)=w231:dbl[])
            n61 = RT FIFO Write(0:w230, 1:w231, 3:w229) -> ()  [unwired: 2 in, 4 out]
            n62 = Split 1D Array(array=w231, index=256) -> (first subarray=→"First FFT (bin)":dbl[], second subarray=→"Second FFT (bin)":dbl[])
            n63 = xnode "Invoke Method"("FPGA VI Reference In"=w237, "error in"=w238, "Number of Elements"=u32 0) -> ("error out"=w239:errorcluster, "Elements Remaining"=→"Elements Remaining FFT":u32)  [unwired: 1 in, 2 out]
          }
        }
      }
      frame #2 {
        n64 = case shown="True" w248 {
          tunnel: w246 -> [w252 w256]
          tunnel: [w252 w257] -> w247
          frame False {
          }
          frame True {
            n65 = Decrement(x="tieni premuto per") -> (x-1=w253:i32)
            n66 = Greater Or Equal?(x=w256, y=w253) -> (x >= y?=w255:bool)
            n67 = case shown="True" w255 {
              tunnel: w256 -> [w258 _]
              tunnel: [w259 0] -> w257
              frame False {
                n68 = Increment(x=w258) -> (x+1=w259:i32)
              }
              frame True {
                n69 = local write "Snapshot"(FALSE ("Snapshot")) -> ()
              }
            }
          }
        }
      }
    }
    n70 = node-c288() -> ()  [unwired: 1 in, 1 out]
  }
  n71 = local read "tieni premuto per"() -> (w8:i32)
  n72 = Add Array Elements(numeric array=w12) -> (sum=w9:dbl)
  n73 = Add Array Elements(numeric array=w11) -> (sum=w10:dbl)
  n74 = Divide(x=w10, y=w8) -> (x/y=→"Mean Noise 2":dbl)
  n75 = Divide(x=w9, y=w8) -> (x/y=→"Mean Noise 1":dbl)
  n76 = node-c288(w32) -> ()  [unwired: 1 out]
  n77 = Merge Errors(w29, w30) -> (w42:errorcluster)
  n78 = flat-sequence {
    tunnel: w42 -> [w268]
    tunnel: w26 -> [w263]
    frame #0 {
      n79 = xnode "Invoke Method"("FPGA VI Reference In"=w263, "error in"=w268) -> ("FPGA VI Reference Out"=w265:refnum<k20>, "error out"=w264:errorcluster)
      n80 = property on="stop" class="Bool (strict)"("Value"=FALSE ("stop")) -> ()  [unwired: 2 in, 2 out]
      n81 = xnode "Invoke Method"("FPGA VI Reference In"=w265, "error in"=w264) -> ("FPGA VI Reference Out"=w266:refnum<k20>, "error out"=w267:errorcluster)
      n82 = xnode "Close FPGA VI Reference"("FPGA VI Reference In"=w266, "error in"=w267) -> ()  [unwired: 1 out]
    }
  }
